vi "Volatus Element.vi"(8 "error in (no error)":errorcluster, 11 "VolatusConfig in":refnum<class "VolatusConfig.lvclass">) -> (0 "error out":errorcluster, 2 "Volatus Element":refnum<class "Config Element.lvclass">, 3 "VolatusConfig out":refnum<class "VolatusConfig.lvclass">)   [LabVIEW 2020, in "VolatusConfig.lvlib" / "VolatusConfig.lvclass"]
uses:
  VolatusConfig.lvclass
  VolatusConfig.lvclass/VolatusConfig.ctl
  lv-cdm/CDM-Config/Config Manager/Config Manager.lvclass
  lv-cdm/CDM-Config/Config Element/Config Element.lvclass
  VolatusConfig.lvlib
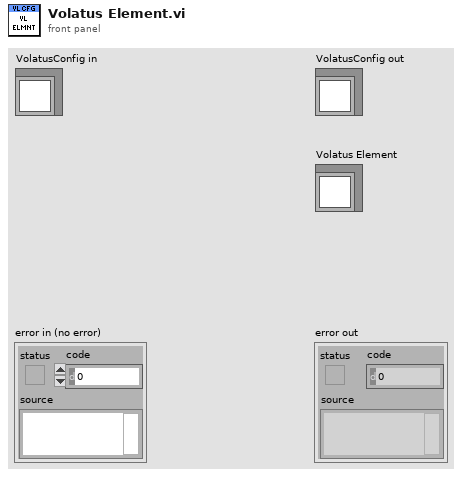
[diagram p1: front panel]
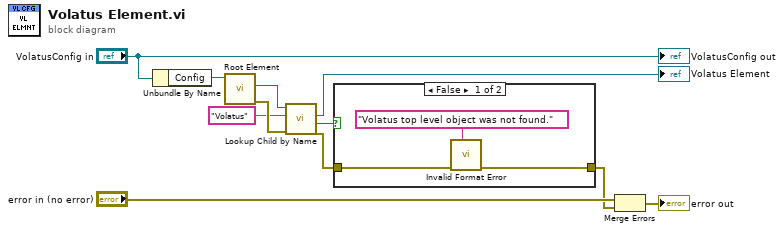
[diagram p0: block diagram]
diagram:
  n1 = Unbundle By Name("VolatusConfig in") -> ("Config"=w9:refnum<class "Config Manager.lvclass">)
  n2 = call "Root Element.vi"("Config Manager in"=w9) -> ("error out"=w10:errorcluster, "Root Element"=w8:refnum<class "Config Element.lvclass">)  [unwired: 8 in, 1 out]
  n3 = call "Lookup Child by Name.vi"("error in (no error)"=w10, "Name"="Volatus", "Config Element in"=w8) -> ("error out"=w3:errorcluster, "Found"=w2:bool, "Child"=→"Volatus Element":refnum<class "Config Element.lvclass">)  [unwired: 5 in, 1 out]
  n4 = case shown="False" w2 {
    tunnel: w3 -> [w13 w15]
    tunnel: [w12 w15] -> w1
    frame False {
      n5 = call "Invalid Format Error.vi"("Context"="Volatus top level object was not found.", "error in (no error)"=w13) -> ("error out"=w12:errorcluster)  [unwired: 9 in]
    }
    frame True {
    }
  }
  n6 = Merge Errors("error in (no error)", w1) -> (→"error out":errorcluster)
  "VolatusConfig out" <- "VolatusConfig in"
